vi "Untitled 3.vi"() -> ()   [LabVIEW 2025]
panel:
  out "Out":bool
  in  "In":bool
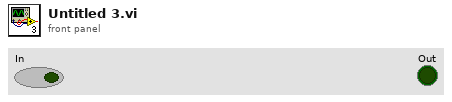
[diagram p1: front panel]
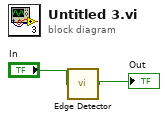
[diagram p0: block diagram]
diagram:
  n1 = call "Edge Detector.vi"("In"="In") -> ("Rising Edge"=→"Out":bool)
